vi "MainCode.vi"() -> ()   [LabVIEW 2023]
uses:
  <extravilib>/ChannelInstances/Tag-bool/Read With Abort.vi
  <extravilib>/ChannelInstances/Tag-bool/Write With Abort.vi
  <vilib>/Instr/_visa.llb/VISA Configure Serial Port (Instr).vi
  <extravilib>/ChannelInstances/Tag-bool/Instantiate.vi
  <extravilib>/ChannelInstances/Tag-bool/EndpointRead.vi
  <vilib>/Utility/file.llb/Write Delimited Spreadsheet (DBL).vi
  <extravilib>/ChannelInstances/Tag-bool/Endpoint.vi
  <extravilib>/ChannelInstances/Tag-bool.lvlib
panel:
  in  "Cooling time":dbl=0.5
  in  "Heating time":dbl=0.5
  out "CO2 concentration ppm":dbl(graph)
  in  "Output massflow":dbl format="%#_13g"
  in  "VISA PID":refnum<visa-resource-name>="COM6"
  out "Mode ON/OFF":bool
  out "Mode PID":bool
  in  "Switch Mode":bool
  in  "DC Pulse (ON/OFF)":bool
  out "Phase indicator":dbl format="%#_13g"
  in  "Sampling time (ms)":dbl format="%#_13g"
  in  "?":path
  in  "Save data":bool
  in  "Input massflow":dbl format="%#_13g"
  in  "C_CO2":dbl format="%#_13g"
  in  "Temp_e_3":dbl format="%#_13g"
  in  "Temp_e_2":dbl format="%#_13g"
  in  "Temp_e_1":dbl format="%#_13g"
  in  "Temp_m_3":dbl format="%#_13g"
  in  "Temp_m_2":dbl format="%#_13g"
  in  "Temp_m_1":dbl format="%#_13g"
  in  "DAC_2_1 (0-10000)":dbl format="%#_13g"
  in  "DAC_2_0 (degrees)":dbl format="%#_13g"
  in  "DAC_1_1 (degrees)":dbl format="%#_13g"
  in  "DAC_1_0 (degrees)":dbl format="%#_13g"
  in  "Current Target Massflow [m^3/h]":dbl format="%#_13g"
  in  "Current Target Temperature [C]":dbl format="%#_13g"
  in  "Start Process":bool
  out "Adsorption":bool
  out "Heating":bool
  out "Desorption":bool
  out "Cooling":bool
  out "Idle":bool
  in  "Stop process":bool
  out "Time elapsed in current phase [s]":dbl
  in  "Adsorption massflow [mV]":dbl
  in  "Adsorption Temperature [C]":dbl
  in  "Desorption massflow [mV]":dbl
  in  "Desorption Temperature  [C]":dbl
  in  "Adsorption Time [Min]":dbl
  in  "Desorption Time [Min]":dbl
  out "Error message parse SCPI":errorcluster
  in  "VISA Arduino":refnum<visa-resource-name>
  in  "STOP PROGRAM":bool
  # "CONTROL PANEL"
  # "SETUP COMMUNICATION"
  # "Process"
  # "For the moment, mass flows under 100m^3/h are not supported"
  # "WARNING: PID arduino cannot communicate on the same port"
  # "Data save path"
  # "For adsorption (90°) and desorption (20°):\n-Adsorption -> 1000mV 208m^3/h\n                            1500mV 307m^3/h\n                            2000mV 406m^3/h\n                            2500mV 505m^3/h\n                            3000mV 604m^3/h\n-Desorption -> 3000mV 200m^3/h \n                           2500mV 180m^3/h \n                           2000mV 130m^3/h \n                           1500mV 100m^3/h\n-Note, these values are subject to change if shit is blocked in front\n-Tested with 3 full columns"
  # "BEFORE ENDING PROGRAM PRESS HERE"
  # "Omega CN740 mode, pulse or PID"
  # "MONITORING"
  # "SENSORS"
  # "ACTUATORS"
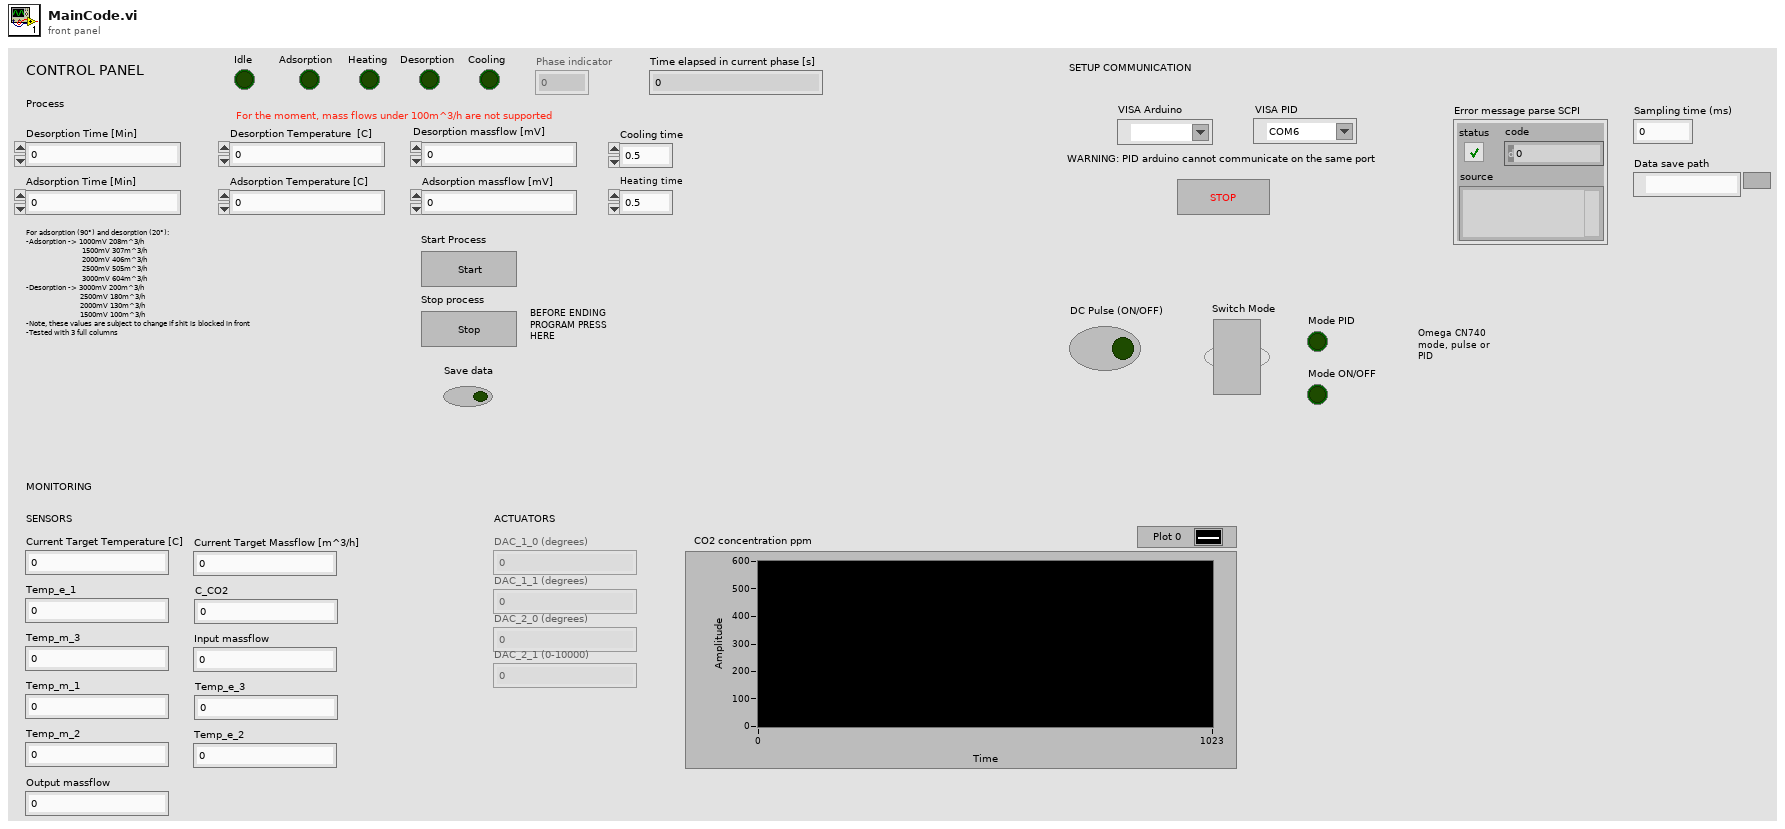
[diagram p1: front panel]
types:
  T1 = typedef "Tag-bool.lvlib/))Channel.ctl" = refnum<queue>
  T2 = cluster{"Temp_m_1":dbl, "Temp_m_2":dbl, "Temp_m_3":dbl, "Temp_e_1":dbl, "Temp_e_2":dbl, "Temp_e_3":dbl, "C_CO2":dbl, "Input massflow":dbl, "Output massflow ":dbl}
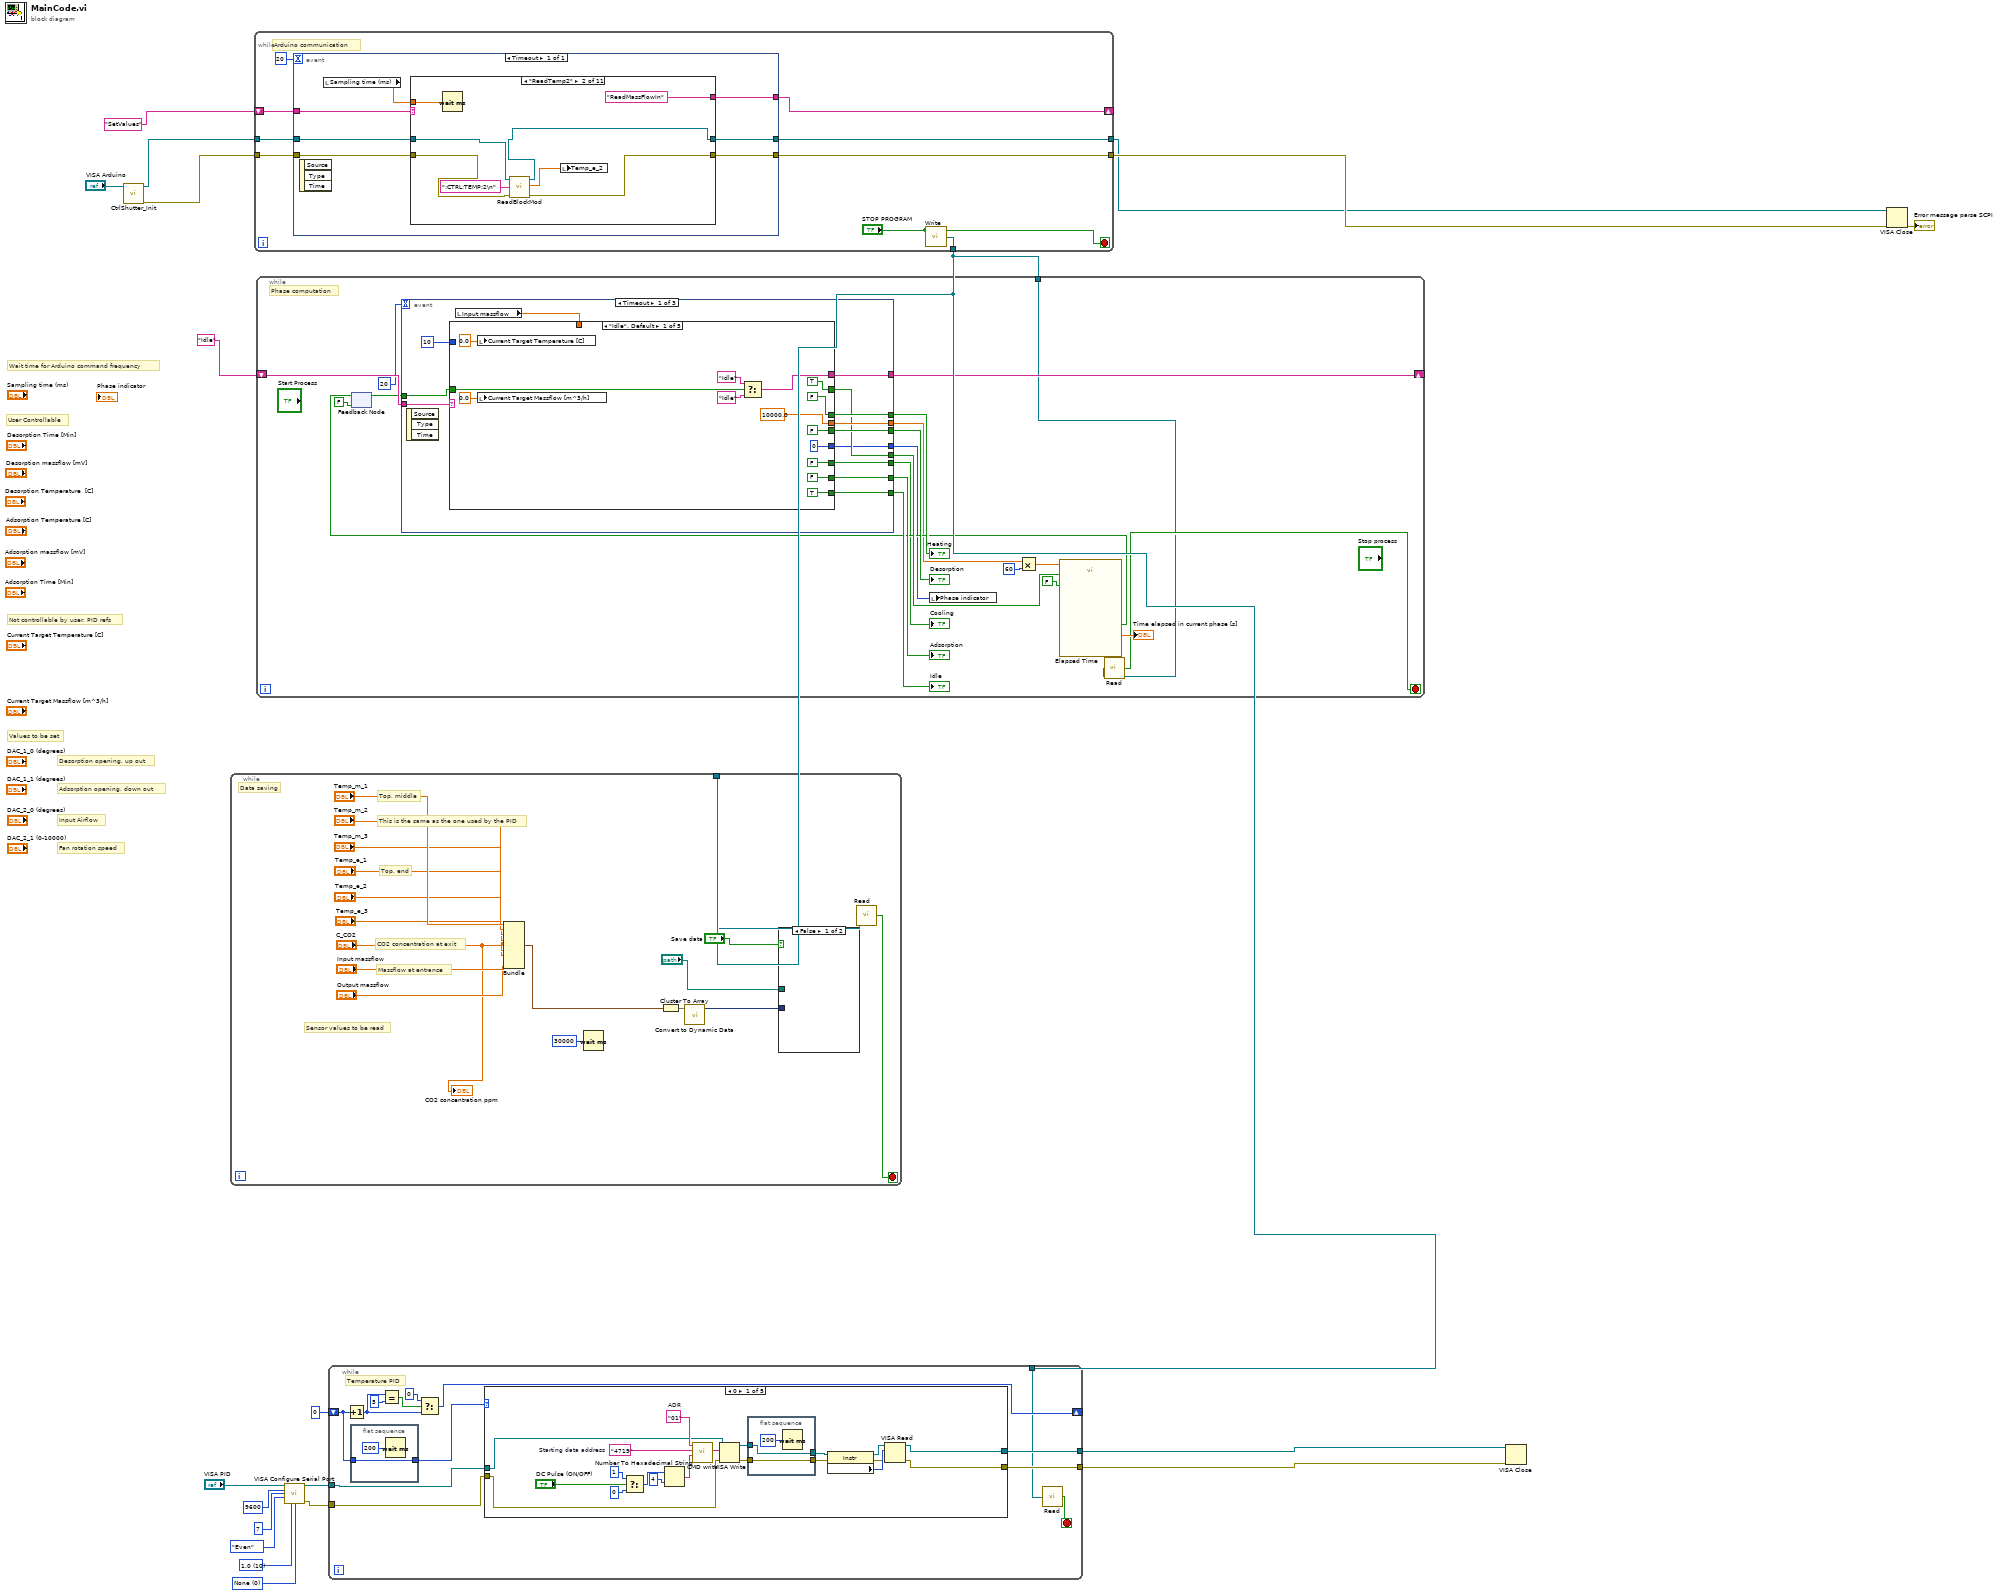
[diagram p0: block diagram]
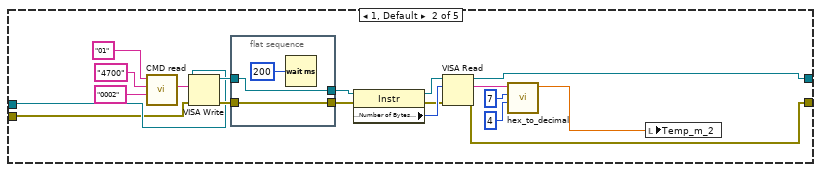
[diagram p2: hidden frame]
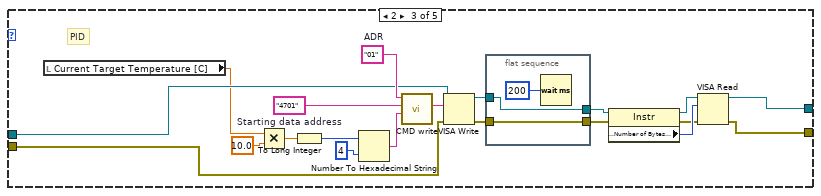
[diagram p3: hidden frame]
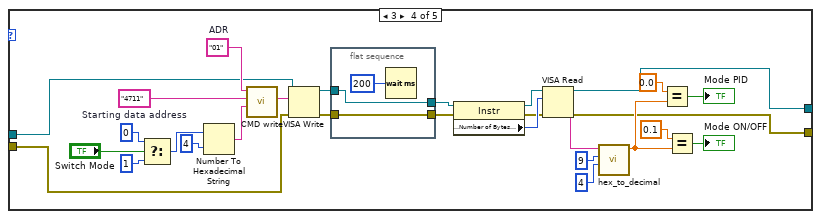
[diagram p4: hidden frame]
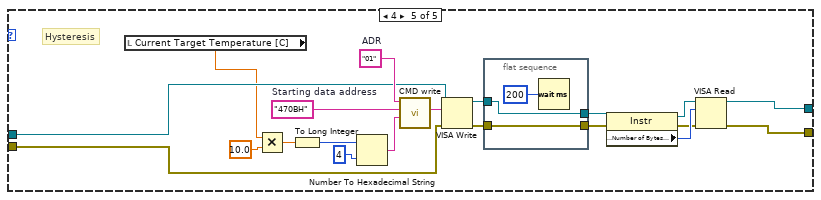
[diagram p5: hidden frame]
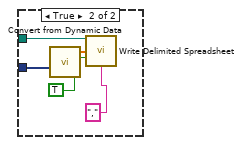
[diagram p6: hidden frame]
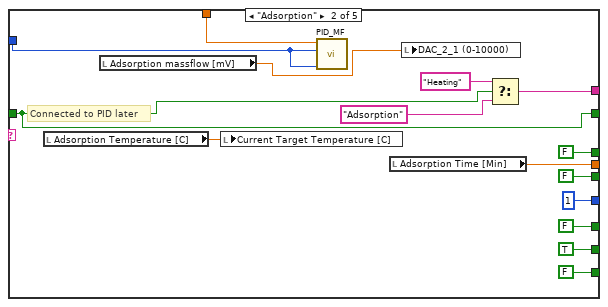
[diagram p7: hidden frame]
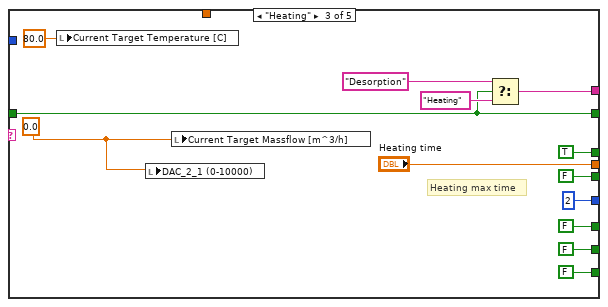
[diagram p8: hidden frame]
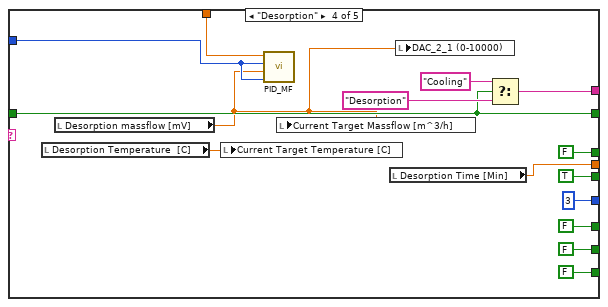
[diagram p9: hidden frame]
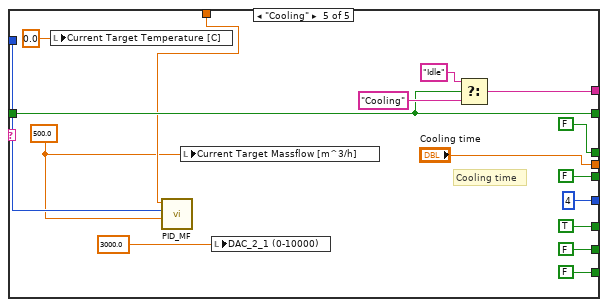
[diagram p10: hidden frame]
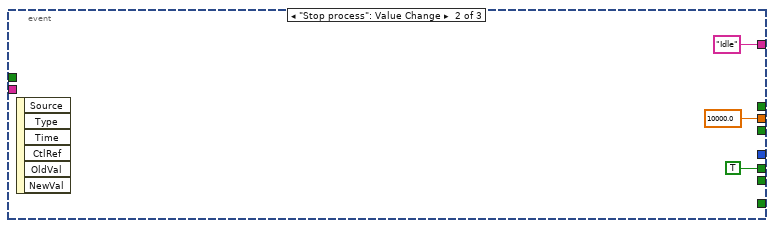
[diagram p11: hidden frame]
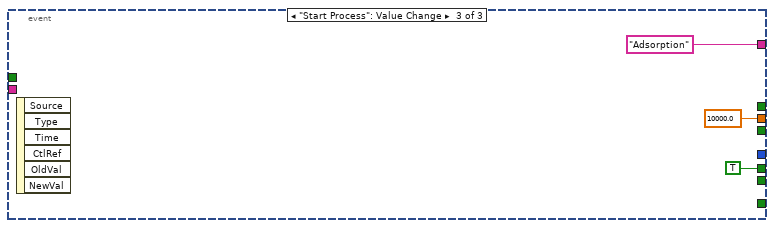
[diagram p12: hidden frame]
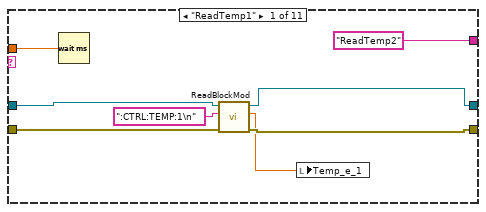
[diagram p13: hidden frame]
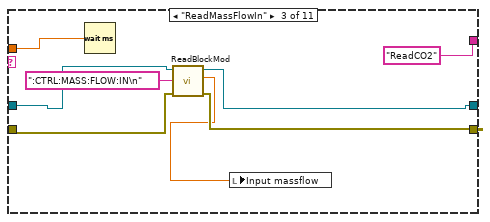
[diagram p14: hidden frame]
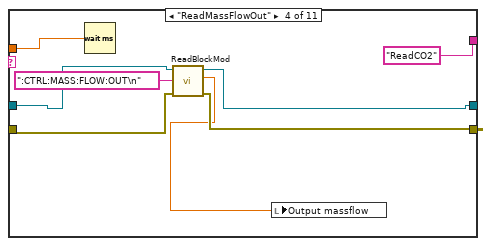
[diagram p15: hidden frame]
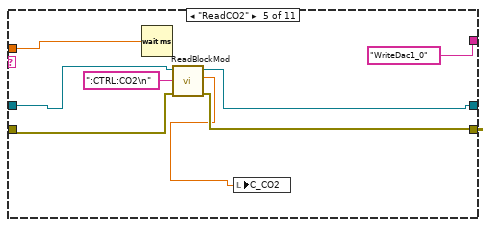
[diagram p16: hidden frame]
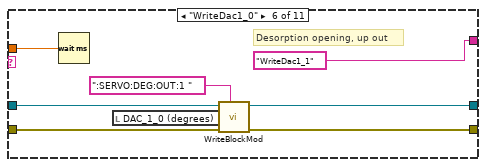
[diagram p17: hidden frame]
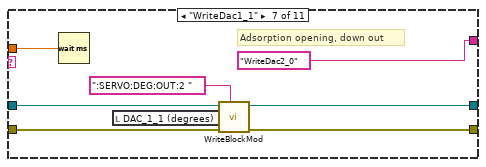
[diagram p18: hidden frame]
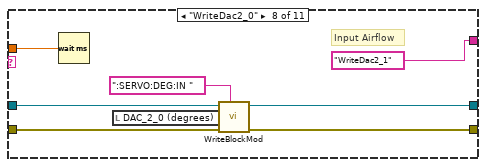
[diagram p19: hidden frame]
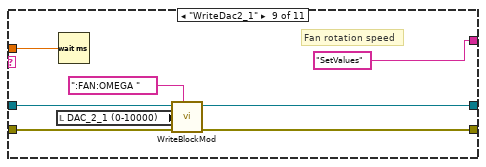
[diagram p20: hidden frame]
diagram:
  w7 = u16 0 items=["None"=0, "XON/XOFF"=1, "RTS/CTS"=2, "DTR/DSR"=4] ("flow control (0:none)")
  w8 = u16 10 items=["1.0"=10, "1.5"=15, "2.0"=20] ("stop bits (10: 1 bit)")
  # "Wait time for Arduino command frequency"
  # "Fan rotation speed"
  # "Input Airflow"
  # "Adsorption opening, down out"
  # "Desorption opening, up out"
  # "Values to be set"
  # "Not controllable by user, PID refs"
  # "User Controllable"
  n1 = call "CtrlShutter_Init.vi"("VISA Refnum in"="VISA Arduino") -> ("error out"=w17:errorcluster, "VISA Refnum out"=w18:refnum<visa-resource-name>)  [unwired: 8 in, 1 out]
  n2 = while {
    tunnel: w18 -> [w28]
    tunnel: w17 -> [w27]
    tunnel: [w26] -> w15
    tunnel: [w25] -> w14
    shift-right: [w23] -> _
    shift-left: "SetValues" ("f") -> [w24]
    tunnel: [w21] -> w1
    stop <- "STOP PROGRAM" stop-if-true
    # "Arduino communication"
    n3 = event shown="[0] Timeout" {
      selector: _ -> [_]
      dyn-events: _ -> [_]
      timeout: 20 -> [_]
      tunnel: [w32] -> w23
      tunnel: w28 -> [w36]
      tunnel: w27 -> [w35]
      tunnel: [w34] -> w26
      tunnel: [w33] -> w25
      tunnel: w24 -> [w31]
      event Timeout {
        n4 = event-data() -> ()  [unwired: 1 in, 3 out]
        n5 = local read "Sampling time (ms)"() -> (w30:dbl)
        n6 = case shown="\"ReadTemp2\"" w31 {
          tunnel: w36 -> [w43 w48 w58 w66 w74 w82 w91 w99 w107 w109 w122]
          tunnel: w35 -> [w42 w49 w54 w63 w71 w78 w90 w98 w106 w110 w123]
          tunnel: [w41 w46 w56 w64 w72 w79 w87 w95 w103 w110 w123] -> w34
          tunnel: [w40 w47 w57 w65 w73 w80 w88 w96 w104 w109 w122] -> w33
          tunnel: ["ReadTemp2" "ReadMassFlowIn" "ReadCO2" "ReadCO2" "WriteDac1_0" "WriteDac1_1" "WriteDac2_0" "WriteDac2_1" "SetValues" "ReadTemp1" "Chillin"] -> w32
          tunnel: w30 -> [w38 w51 w53 w62 w69 w83 w85 w93 w101 w112 _]
          frame "ReadTemp1" {
            n7 = Wait (ms)(milliseconds to wait=w38) -> ()  [unwired: 1 out]
            n8 = call "ReadBlockMod.vi"("VISA Refnum in"=w43, "Command"=":CTRL:TEMP:1\n", "error in (no error)"=w42) -> ("VISA Refnum out"=w40:refnum<visa-resource-name>, "Read value"=w37:dbl, "error out"=w41:errorcluster)  [unwired: 5 in]
            n9 = local write "Temp_e_1"(w37) -> ()
          }
          frame "ReadTemp2" {
            n10 = Wait (ms)(milliseconds to wait=w51) -> ()  [unwired: 1 out]
            n11 = call "ReadBlockMod.vi"("VISA Refnum in"=w48, "Command"=":CTRL:TEMP:2\n", "error in (no error)"=w49) -> ("VISA Refnum out"=w47:refnum<visa-resource-name>, "Read value"=w45:dbl, "error out"=w46:errorcluster)  [unwired: 5 in]
            n12 = local write "Temp_e_2"(w45) -> ()
          }
          frame "ReadMassFlowIn" {
            n13 = Wait (ms)(milliseconds to wait=w53) -> ()  [unwired: 1 out]
            n14 = call "ReadBlockMod.vi"("VISA Refnum in"=w58, "Command"=":CTRL:MASS:FLOW:IN\n", "error in (no error)"=w54) -> ("VISA Refnum out"=w57:refnum<visa-resource-name>, "Read value"=w55:dbl, "error out"=w56:errorcluster)  [unwired: 5 in]
            n15 = local write "Input massflow"(w55) -> ()
          }
          frame "ReadMassFlowOut" {
            n16 = Wait (ms)(milliseconds to wait=w62) -> ()  [unwired: 1 out]
            n17 = call "ReadBlockMod.vi"("VISA Refnum in"=w66, "Command"=":CTRL:MASS:FLOW:OUT\n", "error in (no error)"=w63) -> ("VISA Refnum out"=w65:refnum<visa-resource-name>, "Read value"=w61:dbl, "error out"=w64:errorcluster)  [unwired: 5 in]
            n18 = local write "Output massflow"(w61) -> ()
          }
          frame "ReadCO2" {
            n19 = Wait (ms)(milliseconds to wait=w69) -> ()  [unwired: 1 out]
            n20 = call "ReadBlockMod.vi"("VISA Refnum in"=w74, "Command"=":CTRL:CO2\n", "error in (no error)"=w71) -> ("VISA Refnum out"=w73:refnum<visa-resource-name>, "Read value"=w70:dbl, "error out"=w72:errorcluster)  [unwired: 5 in]
            n21 = local write "C_CO2"(w70) -> ()
          }
          frame "WriteDac1_0" {
            # "Desorption opening, up out"
            n22 = Wait (ms)(milliseconds to wait=w83) -> ()  [unwired: 1 out]
            n23 = local read "DAC_1_0 (degrees)"() -> (w77:dbl)
            n24 = call "WriteBlockMod.vi"("VISA Refnum in"=w82, "Voltage"=w77, "error in (no error)"=w78, "Command"=":SERVO:DEG:OUT:1 ") -> ("VISA Refnum out"=w80:refnum<visa-resource-name>, "error out"=w79:errorcluster)  [unwired: 4 in, 1 out]
          }
          frame "WriteDac1_1" {
            # "Adsorption opening, down out"
            n25 = Wait (ms)(milliseconds to wait=w85) -> ()  [unwired: 1 out]
            n26 = local read "DAC_1_1 (degrees)"() -> (w89:dbl)
            n27 = call "WriteBlockMod.vi"("VISA Refnum in"=w91, "Voltage"=w89, "error in (no error)"=w90, "Command"=":SERVO:DEG:OUT:2 ") -> ("VISA Refnum out"=w88:refnum<visa-resource-name>, "error out"=w87:errorcluster)  [unwired: 4 in, 1 out]
          }
          frame "WriteDac2_0" {
            # "Input Airflow"
            n28 = Wait (ms)(milliseconds to wait=w93) -> ()  [unwired: 1 out]
            n29 = local read "DAC_2_0 (degrees)"() -> (w97:dbl)
            n30 = call "WriteBlockMod.vi"("VISA Refnum in"=w99, "Voltage"=w97, "error in (no error)"=w98, "Command"=":SERVO:DEG:IN ") -> ("VISA Refnum out"=w96:refnum<visa-resource-name>, "error out"=w95:errorcluster)  [unwired: 4 in, 1 out]
          }
          frame "WriteDac2_1" {
            # "Fan rotation speed"
            n31 = local read "DAC_2_1 (0-10000)"() -> (w105:dbl)
            n32 = Wait (ms)(milliseconds to wait=w101) -> ()  [unwired: 1 out]
            n33 = call "WriteBlockMod.vi"("VISA Refnum in"=w107, "Voltage"=w105, "error in (no error)"=w106, "Command"=":FAN:OMEGA ") -> ("VISA Refnum out"=w104:refnum<visa-resource-name>, "error out"=w103:errorcluster)  [unwired: 4 in, 1 out]
          }
          frame "SetValues" {
            n34 = local read "Phase indicator"() -> (w113:dbl)
            n35 = Wait (ms)(milliseconds to wait=w112) -> ()  [unwired: 1 out]
            n36 = case shown="0, Default" w113 {
              frame 0, Default {
                w115 = 90
                # "Idle"
                # "Volts (no direct conversion to mass flow)"
                # "Opening degree"
                n37 = local write "DAC_2_1 (0-10000)"(0) -> ()
                n38 = local write "DAC_1_0 (degrees)"(w115) -> ()
                n39 = local write "DAC_1_1 (degrees)"(w115) -> ()
                n40 = local write "DAC_2_0 (degrees)"(w115) -> ()
              }
              frame 1 {
                (unwired) 0
                w116 = 90
                # "Adsorption"
                # "DAC 2_1 set in phase computation"
                # "closed"
                # "open"
                n41 = local write "DAC_1_0 (degrees)"(0) -> ()
                n42 = local write "DAC_1_1 (degrees)"(w116) -> ()
                n43 = local write "DAC_2_0 (degrees)"(w116) -> ()
              }
              frame 2 {
                (unwired) 0
                w118 = 0
                # "Heating"
                # "closed"
                n44 = local write "DAC_1_0 (degrees)"(w118) -> ()
                n45 = local write "DAC_1_1 (degrees)"(w118) -> ()
                n46 = local write "DAC_2_0 (degrees)"(w118) -> ()
              }
              frame 3 {
                (unwired) 20
                w119 = 90
                (unwired) 0
                # "Desorption"
                # "closed"
                n47 = local write "DAC_1_0 (degrees)"(w119) -> ()
                n48 = local write "DAC_1_1 (degrees)"(0) -> ()
                n49 = local write "DAC_2_0 (degrees)"(w119) -> ()
              }
              frame 4 {
                w121 = 90
                # "Cooling"
                # "closed"
                n50 = local write "DAC_1_0 (degrees)"(w121) -> ()
                n51 = local write "DAC_1_1 (degrees)"(w121) -> ()
                n52 = local write "DAC_2_0 (degrees)"(w121) -> ()
              }
            }
          }
          frame "Chillin", Default {
          }
        }
      }
    }
    n53 = call <extravilib>:"Write.vi"("element"="STOP PROGRAM") -> ("channel"=w21:T1)  [unwired: 1 out]
  }
  n54 = while {
    tunnel: w1 -> [w138]
    stop <- w141 stop-if-true
    # "Massflow at entrance"
    # "CO2 concentration at exit"
    # "Top, end"
    # "This is the same as the one used by the PID"
    # "Top, middle"
    # "Sensor values to be read"
    # "Data saving"
    n55 = Bundle("Temp_m_1"="Temp_m_1", "Temp_m_2"="Temp_m_2", "Temp_m_3"="Temp_m_3", "Temp_e_1"="Temp_e_1", "Temp_e_2"="Temp_e_2", "Temp_e_3"="Temp_e_3", "C_CO2"="C_CO2", "Input massflow"="Input massflow", "Output massflow"="Output massflow") -> (w127:T2)  [unwired: 1 in]
    n56 = Wait (ms)(milliseconds to wait=u32 30000) -> ()  [unwired: 1 out]
    n57 = Cluster To Array(cluster=w127) -> (array=w139:dbl[])
    n58 = call "Convert to Dynamic Data"("Array"=w139) -> ("Dynamic Data Type"=w137:dynamicdata)  [unwired: 3 in]
    n59 = case shown="False" "Save data" {
      tunnel: w137 -> [_ w146]
      tunnel: "?" -> [_ w144]
      frame False {
      }
      frame True {
        n60 = call "Convert from Dynamic Data"("Dynamic Data Type"=w146) -> ("Array"=w145:dbl[])  [unwired: 3 in]
        n61 = call-poly <vilib>:"Write Delimited Spreadsheet.vi"("file path (dialog if empty)"=w144, "1D data"=w145, "append to file? (new file:F)"=TRUE, "delimiter (\\t)"=",") -> ()  [unwired: 10 in, 2 out]
      }
    }
    n62 = call <extravilib>:"Read.vi"("channel"=w138) -> ("element"=w141:bool)  [unwired: 1 in, 1 out]
    "CO2 concentration ppm" <- "C_CO2"
  }
  n63 = while {
    shift-right: [w160] -> _
    shift-left: "Idle" ("f") -> [w159]
    tunnel: w1 -> [w151]
    stop <- w152 stop-if-true
    # "Phase computation"
    n64 = feedback #1(FALSE) -> (w156:bool)
    n65 = event shown="[0] Timeout" {
      selector: _ -> [_ _ _]
      dyn-events: _ -> [_ _ _]
      timeout: 20 -> [_ _ _]
      tunnel: [w179 _ _] -> w166
      tunnel: [w178 _ _] -> w165
      tunnel: [w177 _ _] -> w164
      tunnel: [w176 _ _] -> w163
      tunnel: [w175 _ _] -> w153
      tunnel: [w174 10000.0 10000.0] -> w148
      tunnel: [w173 TRUE TRUE] -> w162
      tunnel: w156 -> [w172 _ _]
      tunnel: [w170 "Idle" ("f") "Adsorption" ("f")] -> w160
      tunnel: w159 -> [w171 _ _]
      tunnel: [w169 _ _] -> w150
      event Timeout {
        n66 = event-data() -> ()  [unwired: 1 in, 3 out]
        n67 = local read "Input massflow"() -> (w168:dbl)
        n68 = case shown="\"Idle\", Default" w171 {
          tunnel: [w186 w203 w214 w229 w246] -> w170
          tunnel: [TRUE FALSE FALSE FALSE FALSE] -> w179
          tunnel: [FALSE TRUE FALSE FALSE FALSE] -> w178
          tunnel: [FALSE FALSE TRUE FALSE FALSE] -> w177
          tunnel: [FALSE FALSE FALSE TRUE FALSE] -> w176
          tunnel: [FALSE FALSE FALSE FALSE TRUE] -> w175
          tunnel: [10000.0 w199 "Heating time" w227 "Cooling time"] -> w174
          tunnel: [TRUE w201 w213 w228 w244] -> w173
          tunnel: w172 -> [w183 w201 w213 w228 w244]
          tunnel: [0 1 2 3 4] -> w169
          tunnel: w168 -> [_ w196 _ w223 w241]
          tunnel: 10 -> [_ w195 _ w224 w240]
          frame "Idle", Default {
            n69 = local write "Current Target Temperature [C]"(0.0) -> ()
            n70 = local write "Current Target Massflow [m^3/h]"(0.0) -> ()
            n71 = Select(t="Idle", s=w183, f="Idle") -> (s? t:f=w186:string)
          }
          frame "Adsorption" {
            # "Connected to PID later"
            n72 = local read "Adsorption Temperature [C]"() -> (w197:dbl)
            n73 = local read "Adsorption massflow [mV]"() -> (w194:dbl)
            n74 = local write "Current Target Temperature [C]"(w197) -> ()
            n75 = call "PID_MF.vi"("Time to wait between updates B  (ms)"=w195, "Time to wait between updates A  (ms)"=w195, "Real massflow"=w196) -> ()  [unwired: 7 in, 2 out]
            n76 = local read "Adsorption Time [Min]"() -> (w199:dbl)
            n77 = local write "DAC_2_1 (0-10000)"(w194) -> ()
            n78 = Select(t="Heating", s=w201, f="Adsorption") -> (s? t:f=w203:string)
          }
          frame "Heating" {
            w210 = 0.0
            # "Heating max time"
            n79 = local write "Current Target Temperature [C]"(80.0) -> ()
            n80 = local write "DAC_2_1 (0-10000)"(w210) -> ()
            n81 = local write "Current Target Massflow [m^3/h]"(w210) -> ()
            n82 = Select(t="Desorption", s=w213, f="Heating") -> (s? t:f=w214:string)
          }
          frame "Desorption" {
            n83 = local read "Desorption Temperature  [C]"() -> (w226:dbl)
            n84 = local read "Desorption massflow [mV]"() -> (w222:dbl)
            n85 = local write "Current Target Temperature [C]"(w226) -> ()
            n86 = call "PID_MF.vi"("Time to wait between updates B  (ms)"=w224, "Target Massflow"=w222, "Time to wait between updates A  (ms)"=w224, "Real massflow"=w223) -> ()  [unwired: 6 in, 2 out]
            n87 = local write "Current Target Massflow [m^3/h]"(w222) -> ()
            n88 = local read "Desorption Time [Min]"() -> (w227:dbl)
            n89 = local write "DAC_2_1 (0-10000)"(w222) -> ()
            n90 = Select(t="Cooling", s=w228, f="Desorption") -> (s? t:f=w229:string)
          }
          frame "Cooling" {
            w239 = 500.0
            # "Cooling time"
            n91 = local write "Current Target Temperature [C]"(0.0) -> ()
            n92 = call "PID_MF.vi"("Target Massflow"=w239, "Time to wait between updates A  (ms)"=w240, "Real massflow"=w241) -> ()  [unwired: 7 in, 2 out]
            n93 = local write "Current Target Massflow [m^3/h]"(w239) -> ()
            n94 = local write "DAC_2_1 (0-10000)"(3000.0) -> ()
            n95 = Select(t="Idle", s=w244, f="Cooling") -> (s? t:f=w246:string)
          }
        }
      }
      event "Stop process": Value Change {
        n96 = event-data() -> ()  [unwired: 1 in, 6 out]
      }
      event "Start Process": Value Change {
        n97 = event-data() -> ()  [unwired: 1 in, 6 out]
      }
    }
    "Adsorption" <- w165
    "Heating" <- w164
    "Desorption" <- w163
    "Cooling" <- w153
    "Idle" <- w166
    n98 = local write "Phase indicator"(w150) -> ()
    n99 = Multiply(x=w148, y=60) -> (x*y=w147:dbl)
    n100 = call "Elapsed Time"("Time Target (s)"=w147, "Reset"=w162, "Auto Reset"=FALSE) -> ("Elapsed Time (s)"=→"Time elapsed in current phase [s]":dbl, "Time has Elapsed"=w157:bool)  [unwired: 9 in, 6 out]
    n101 = feedback-in #1(w157) -> ()
    n102 = call <extravilib>:"Read.vi"("channel"=w151) -> ("element"=w152:bool)  [unwired: 1 in, 1 out]
  }
  n103 = call-poly "VISA Configure Serial Port"("VISA resource name"="VISA PID", "baud rate (9600)"=u32 9600, "data bits (8)"=u16 7, "parity (0:none)"=enum16{"None", "Odd", "Even", "Mark", "Space"}."Even", "stop bits (10: 1 bit)"=w8, "flow control (0:none)"=w7) -> ("VISA resource name out"=w6:refnum<visa-resource-name>, "error out"=w5:errorcluster)  [unwired: 2 in, 6 out]
  n104 = while {
    tunnel: w6 -> [w266]
    tunnel: w5 -> [w265]
    shift-right: [w263] -> _
    shift-left: 0 -> [w264]
    tunnel: [w262] -> w3
    tunnel: [w261] -> w2
    tunnel: w1 -> [w259]
    stop <- w260 stop-if-true
    # "Temperature PID"
    n105 = Increment(x=w264) -> (x+1=w269:i32)
    n106 = flat-sequence {
      tunnel: w264 -> [w272]
      tunnel: [w272] -> w267
      frame #0 {
        n107 = Wait (ms)(milliseconds to wait=u32 200 ("attente (ms)")) -> ()  [unwired: 1 out]
      }
    }
    n108 = Equal?(x=w269, y=5) -> (x = y?=w270:bool)
    n109 = Select(t=0, s=w270, f=w269) -> (s? t:f=w263:i32)
    n110 = case shown="0" w267 {
      tunnel: w266 -> [w277 w301 w323 w354 w377]
      tunnel: w265 -> [w276 w300 w322 w353 w376]
      tunnel: [w275 w299 w321 w343 w375] -> w262
      tunnel: [w274 w298 w320 w342 w374] -> w261
      frame 0 {
        w286 = "01"  # ADR
        w285 = "4719"  # Starting data address
        n111 = Select(t=1, s="DC Pulse (ON/OFF)", f=0) -> (s? t:f=w280:i32)
        n112 = Number To Hexadecimal String(1:i16 4 ("largeur (-)"), 2:w280) -> (0:w278:string)
        n113 = call "CMD write.vi"("Data Content"=w278, "Starting data address"=w285, "ADR"=w286) -> ("Chaîne en sortie"=w284:string)  [unwired: 6 in]
        n114 = VISA Write(VISA resource name=w277, write buffer=w284, error in (no error)=w276) -> (VISA resource name out=w290:refnum<visa-resource-name>, error out=w287:errorcluster)  [unwired: 1 out]
        n115 = flat-sequence {
          tunnel: w290 -> [w295]
          tunnel: [w295] -> w289
          tunnel: [w294] -> w288
          tunnel: w287 -> [w294]
          frame #0 {
            n116 = Wait (ms)(milliseconds to wait=u32 200 ("attente (ms)")) -> ()  [unwired: 1 out]
          }
        }
        n117 = property class="Instr"(reference=w289, error in=w288) -> (reference out=w293:refnum<visa-resource-name>, error out=w291:errorcluster, "Serial Settings:Number of Bytes at Serial Port"=w292:u32)
        n118 = VISA Read(VISA resource name=w293, byte count=w292, error in (no error)=w291) -> (VISA resource name out=w275:refnum<visa-resource-name>, error out=w274:errorcluster)  [unwired: 2 out]
      }
      frame 1, Default {
        n119 = call "CMD read.vi"("Data Content"="0002", "Starting data address"="4700", "ADR"="01") -> ("Chaîne en sortie"=w303:string)  [unwired: 6 in]
        n120 = VISA Write(VISA resource name=w301, write buffer=w303, error in (no error)=w300) -> (VISA resource name out=w312:refnum<visa-resource-name>, error out=w309:errorcluster)  [unwired: 1 out]
        n121 = flat-sequence {
          tunnel: w312 -> [w317]
          tunnel: [w317] -> w311
          tunnel: [w316] -> w310
          tunnel: w309 -> [w316]
          frame #0 {
            n122 = Wait (ms)(milliseconds to wait=u32 200 ("attente (ms)")) -> ()  [unwired: 1 out]
          }
        }
        n123 = property class="Instr"(reference=w311, error in=w310) -> (reference out=w315:refnum<visa-resource-name>, error out=w313:errorcluster, "Serial Settings:Number of Bytes at Serial Port"=w314:u32)
        n124 = VISA Read(VISA resource name=w315, byte count=w314, error in (no error)=w313) -> (VISA resource name out=w299:refnum<visa-resource-name>, read buffer=w302:string, error out=w298:errorcluster)  [unwired: 1 out]
        n125 = call "hex_to_decimal.vi"("length (rest)"=4, "offset (0)"=7, "read buffer"=w302) -> ("Numeric"=w297:dbl)  [unwired: 8 in]
        n126 = local write "Temp_m_2"(w297) -> ()
      }
      frame 2 {
        w327 = "01"  # ADR
        w325 = "4701"  # Starting data address
        # "PID"
        n127 = local read "Current Target Temperature [C]"() -> (w319:dbl)
        n128 = Multiply(x=w319, y=10.0) -> (x*y=w335:dbl)
        n129 = To Long Integer(number=w335) -> (32bit integer=w338:i32)
        n130 = Number To Hexadecimal String(1:i16 4 ("largeur (-)"), 2:w338) -> (0:w326:string)
        n131 = call "CMD write.vi"("Data Content"=w326, "Starting data address"=w325, "ADR"=w327) -> ("Chaîne en sortie"=w324:string)  [unwired: 6 in]
        n132 = VISA Write(VISA resource name=w323, write buffer=w324, error in (no error)=w322) -> (VISA resource name out=w331:refnum<visa-resource-name>, error out=w328:errorcluster)  [unwired: 1 out]
        n133 = flat-sequence {
          tunnel: w331 -> [w340]
          tunnel: [w340] -> w330
          tunnel: [w339] -> w329
          tunnel: w328 -> [w339]
          frame #0 {
            n134 = Wait (ms)(milliseconds to wait=u32 200 ("attente (ms)")) -> ()  [unwired: 1 out]
          }
        }
        n135 = property class="Instr"(reference=w330, error in=w329) -> (reference out=w334:refnum<visa-resource-name>, error out=w332:errorcluster, "Serial Settings:Number of Bytes at Serial Port"=w333:u32)
        n136 = VISA Read(VISA resource name=w334, byte count=w333, error in (no error)=w332) -> (VISA resource name out=w321:refnum<visa-resource-name>, error out=w320:errorcluster)  [unwired: 2 out]
      }
      frame 3 {
        w362 = "01"  # ADR
        w361 = "4711"  # Starting data address
        n137 = Select(t=0, s="Switch Mode", f=1) -> (s? t:f=w357:i32)
        n138 = Number To Hexadecimal String(1:i16 4 ("largeur (-)"), 2:w357) -> (0:w355:string)
        n139 = call "CMD write.vi"("Data Content"=w355, "Starting data address"=w361, "ADR"=w362) -> ("Chaîne en sortie"=w360:string)  [unwired: 6 in]
        n140 = VISA Write(VISA resource name=w354, write buffer=w360, error in (no error)=w353) -> (VISA resource name out=w366:refnum<visa-resource-name>, error out=w363:errorcluster)  [unwired: 1 out]
        n141 = flat-sequence {
          tunnel: w366 -> [w371]
          tunnel: [w371] -> w365
          tunnel: [w370] -> w364
          tunnel: w363 -> [w370]
          frame #0 {
            n142 = Wait (ms)(milliseconds to wait=u32 200 ("attente (ms)")) -> ()  [unwired: 1 out]
          }
        }
        n143 = property class="Instr"(reference=w365, error in=w364) -> (reference out=w369:refnum<visa-resource-name>, error out=w367:errorcluster, "Serial Settings:Number of Bytes at Serial Port"=w368:u32)
        n144 = VISA Read(VISA resource name=w369, byte count=w368, error in (no error)=w367) -> (VISA resource name out=w343:refnum<visa-resource-name>, read buffer=w350:string, error out=w342:errorcluster)  [unwired: 1 out]
        n145 = call "hex_to_decimal.vi"("length (rest)"=4, "offset (0)"=9, "read buffer"=w350) -> ("Numeric"=w348:dbl)  [unwired: 8 in]
        n146 = Equal?(x=0.0, y=w348) -> (x = y?=→"Mode PID":bool)
        n147 = Equal?(x=0.1, y=w348) -> (x = y?=→"Mode ON/OFF":bool)
      }
      frame 4 {
        w381 = "01"  # ADR
        w379 = "470BH"  # Starting data address
        # "Hysteresis"
        n148 = local read "Current Target Temperature [C]"() -> (w373:dbl)
        n149 = Multiply(x=w373, y=10.0) -> (x*y=w389:dbl)
        n150 = To Long Integer(number=w389) -> (32bit integer=w392:i32)
        n151 = Number To Hexadecimal String(1:i16 4 ("largeur (-)"), 2:w392) -> (0:w380:string)
        n152 = call "CMD write.vi"("Data Content"=w380, "Starting data address"=w379, "ADR"=w381) -> ("Chaîne en sortie"=w378:string)  [unwired: 6 in]
        n153 = VISA Write(VISA resource name=w377, write buffer=w378, error in (no error)=w376) -> (VISA resource name out=w385:refnum<visa-resource-name>, error out=w382:errorcluster)  [unwired: 1 out]
        n154 = flat-sequence {
          tunnel: w385 -> [w394]
          tunnel: [w394] -> w384
          tunnel: [w393] -> w383
          tunnel: w382 -> [w393]
          frame #0 {
            n155 = Wait (ms)(milliseconds to wait=u32 200 ("attente (ms)")) -> ()  [unwired: 1 out]
          }
        }
        n156 = property class="Instr"(reference=w384, error in=w383) -> (reference out=w388:refnum<visa-resource-name>, error out=w386:errorcluster, "Serial Settings:Number of Bytes at Serial Port"=w387:u32)
        n157 = VISA Read(VISA resource name=w388, byte count=w387, error in (no error)=w386) -> (VISA resource name out=w375:refnum<visa-resource-name>, error out=w374:errorcluster)  [unwired: 2 out]
      }
    }
    n158 = call <extravilib>:"Read.vi"("channel"=w259) -> ("element"=w260:bool)  [unwired: 1 in, 1 out]
  }
  n159 = VISA Close(VISA resource name=w3, error in (no error)=w2) -> ()  [unwired: 1 out]
  n160 = VISA Close(VISA resource name=w14, error in (no error)=w15) -> (error out=→"Error message parse SCPI":errorcluster)
